vi "Windspeed Warnings.vi"(8 "error in":errorcluster, 10 "Max Windspeed":dbl, 11 "Current Windspeed":dbl) -> (0 "error out":errorcluster, 2 "Windspeed Warning Text":string="No Warning", 3 "Windspeed Warning?":bool)   [LabVIEW 2013]
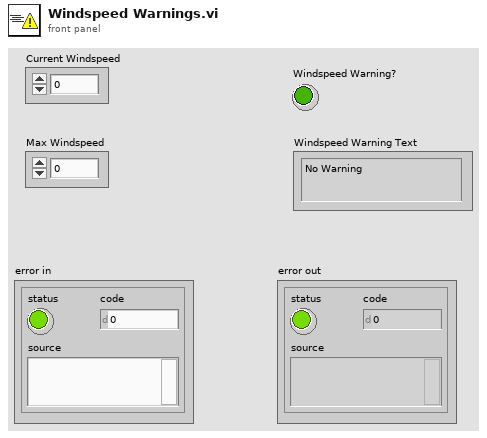
[diagram p1: front panel]
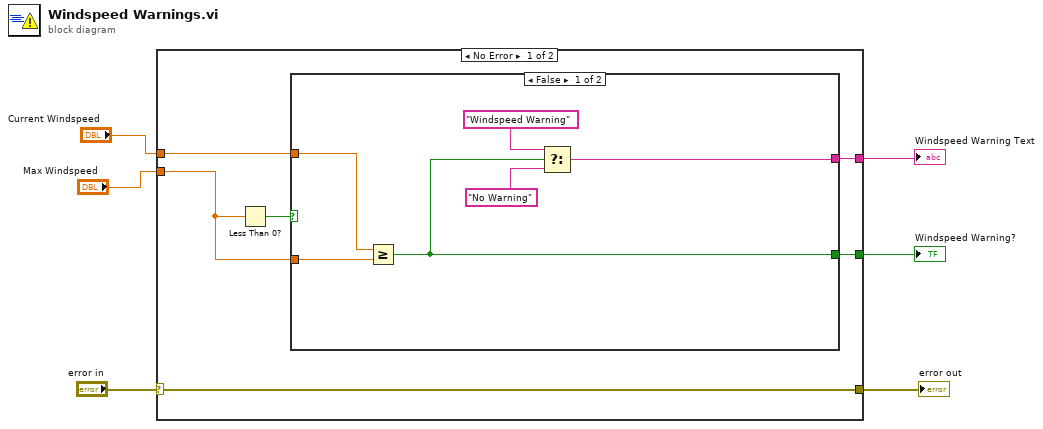
[diagram p0: block diagram]
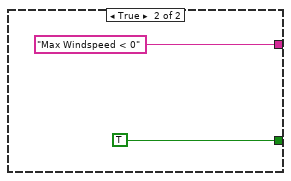
[diagram p2: hidden frame]
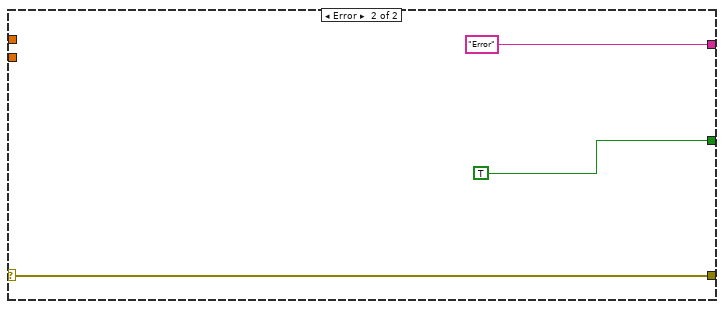
[diagram p3: hidden frame]
diagram:
  n1 = case shown="No Error" "error in" {
    selector: "error in" -> [w9 w23]
    tunnel: [w12 "Error" ("f")] -> w1
    tunnel: [w11 TRUE] -> w2
    tunnel: [w9 w23] -> w5
    tunnel: "Current Windspeed" -> [w8 _]
    tunnel: "Max Windspeed" -> [w7 _]
    frame No Error {
      n2 = Less Than 0?(x=w7) -> (x < 0?=w10:bool)
      n3 = case shown="False" w10 {
        tunnel: [w14 "Max Windspeed < 0" ("f")] -> w12
        tunnel: [w13 TRUE] -> w11
        tunnel: w7 -> [w18 _]
        tunnel: w8 -> [w15 _]
        frame False {
          n4 = Greater Or Equal?(x=w15, y=w18) -> (x >= y?=w13:bool)
          n5 = Select(t="Windspeed Warning", s=w13, f="No Warning") -> (s? t:f=w14:string)
        }
        frame True {
        }
      }
    }
    frame Error {
    }
  }
  "error out" <- w5
  "Windspeed Warning?" <- w2
  "Windspeed Warning Text" <- w1
